vi "Test VI.vi"() -> ()   [LabVIEW 2014]
uses:
  <vilib>/Utility/tdmsutil.llb/TDMS Generate Random Data (DBL).vi
panel:
  out "Table":string[][](table)
  in  "Buffer Size":i32=100000 format="%.0p"
  in  "Folder":path=path "C:/Ehsan Temp Folder/TFS/LV/Data Logging with LabVIEW/Good Examples/TDMS Best Practices 2010 (3)"
  in  "chunk size":i32=1000 format="%.0p"
  in  "number of samples":i32=10000000 format="%.0p"
  # "Number of Samples: Total amount of data (x2) to be generated and written to file.\nChunk Size: Number of samples to write each iteration\nBuffer Size: For the buffer method, the size of the buffer.  This will produce an effective chunk size so if they match we expect similar results.\nFile Compression: Size of the file relative to the size of the data. i.e. 100% is a pure binary file, 150% means for every 1MB data there is 1.5MB file.\n                                 This gives a good indication of the framentation of a file.  The larger this is, the more fragmented and the worse read performance."
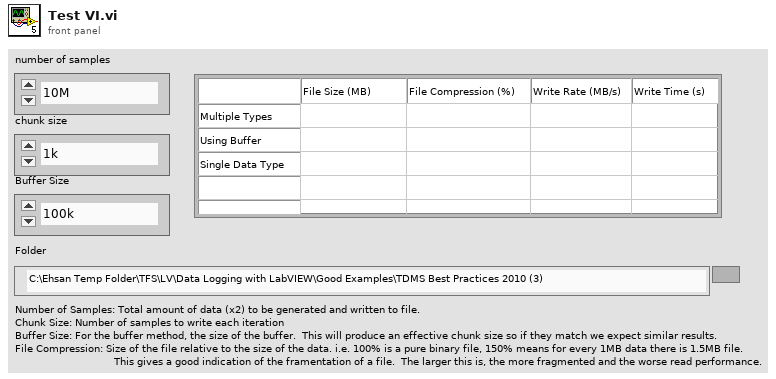
[diagram p1: front panel]
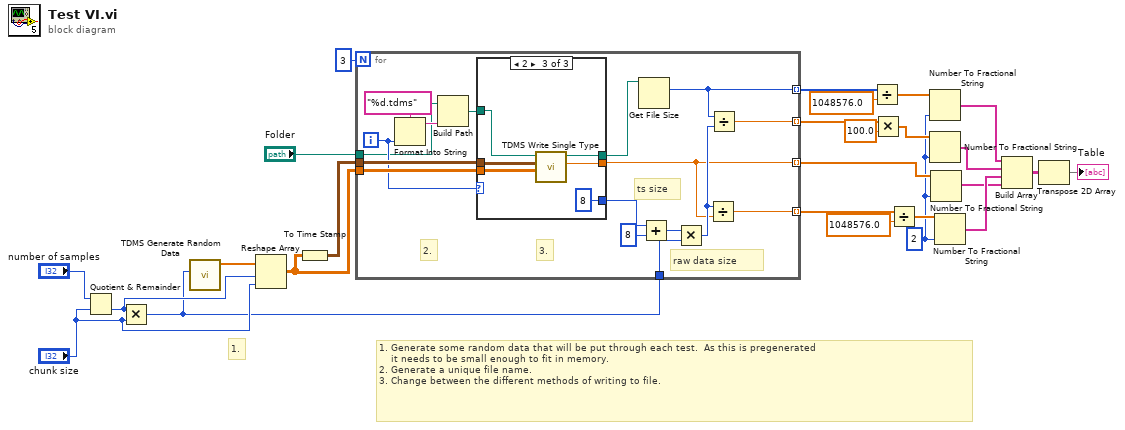
[diagram p0: block diagram]
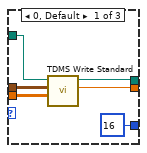
[diagram p2: hidden frame]
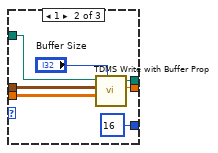
[diagram p3: hidden frame]
diagram:
  w1 = i16 2 ("precision (6)")
  # "1. Generate some random data that will be put through each test.  As this is pregenerated\n    it needs to be small enough to fit in memory.\n2. Generate a unique file name.\n3. Change between the different methods of writing to file."
  # "1."
  n1 = Quotient & Remainder(x="number of samples", y="chunk size") -> (floor(x/y)=w20:i32)  [unwired: 1 out]
  n2 = Multiply(x=w20, y="chunk size") -> (x*y=w19:i32)
  n3 = call-poly <vilib>:"TDMS Generate Random Data.vi"("number of samples"=w19) -> ("data"=w25:dbl[])  [unwired: 9 in, 1 out]
  n4 = Reshape Array(w25, w20, "chunk size") -> (w23:dbl[][])
  n5 = To Time Stamp(1:w23) -> (0:w24:timestamp[][])
  n6 = for {
    N: 3 -> [_]
    tunnel: w24 -> [w43]
    tunnel: w23 -> [w42]
    tunnel: "Folder" -> [w36]
    tunnel: w19 -> [w32]
    tunnel: [w31] -> w17 mode=indexing
    tunnel: [w29] -> w6 mode=indexing
    tunnel: [w28] -> w13 mode=indexing
    tunnel: [w27] -> w12 mode=indexing
    i -> [w37]
    # "3."
    # "2."
    # "raw data size"
    # "ts size"
    n7 = Format Into String(format string="%d.tdms", w37) -> (resulting string=w39:string)  [unwired: 2 in, 1 out]
    n8 = Build Path(base path=w36, name or relative path=w39) -> (appended path=w38:path)
    n9 = case shown="2" w37 {
      tunnel: w43 -> [w49 w56 w61]
      tunnel: w42 -> [w48 w55 w60]
      tunnel: [w46 w54 w59] -> w29
      tunnel: [w47 w53 w62] -> w41
      tunnel: w38 -> [w44 w51 w57]
      tunnel: [16 16 8] -> w35
      frame 0, Default {
        n10 = call "TDMS Write Standard.vi"("Data"=w48, "Timestamps"=w49, "Path"=w44) -> ("Time for Write (S)"=w46:dbl, "Path Out"=w47:path)  [unwired: 6 in, 1 out]
      }
      frame 1 {
        n11 = call "TDMS Write with Buffer Prop.vi"("Buffer Size"="Buffer Size", "Data"=w55, "Timestamps"=w56, "Path"=w51) -> ("Time for Write (S)"=w54:dbl, "Path Out"=w53:path)  [unwired: 5 in, 1 out]
      }
      frame 2 {
        n12 = call "TDMS Write Single Type.vi"("Data"=w60, "Timestamps"=w61, "Path"=w57) -> ("Time for Write (S)"=w59:dbl, "Path Out"=w62:path)  [unwired: 6 in, 1 out]
      }
    }
    n13 = Get File Size(file=w41) -> (size (in bytes)=w27:i64)  [unwired: 1 in, 2 out]
    n14 = Add(x=w35, y=8) -> (x+y=w33:i32)
    n15 = Multiply(x=w33, y=w32) -> (x*y=w30:i32)
    n16 = Divide(x=w30, y=w29) -> (x/y=w31:dbl)
    n17 = Divide(x=w27, y=w30) -> (x/y=w28:dbl)
  }
  n18 = Divide(x=w12, y=1048576.0) -> (x/y=w11:dbl[])
  n19 = Multiply(x=w13, y=100.0) -> (x*y=w10:dbl[])
  n20 = Divide(x=w17, y=1048576.0) -> (x/y=w9:dbl[])
  n21 = Number To Fractional String(number=w11, precision (6)=w1) -> (F-format string=w8:string[])  [unwired: 2 in]
  n22 = Number To Fractional String(number=w10, precision (6)=w1) -> (F-format string=w7:string[])  [unwired: 2 in]
  n23 = Number To Fractional String(number=w6, precision (6)=w1) -> (F-format string=w4:string[])  [unwired: 2 in]
  n24 = Number To Fractional String(number=w9, precision (6)=w1) -> (F-format string=w5:string[])  [unwired: 2 in]
  n25 = Build Array(w8, w7, w5, w4) -> (w3:string[][])
  n26 = Transpose 2D Array(2D array=w3) -> (transposed array=→"Table":string[][])
